vi "LSX Set Dig IO Distance.vi"(6 "lAxis":i32, 7 "dDist":dbl, 8 "error in (no error)":errorcluster, 9 "bFkt":i32, 10 "lIndex":i32, 11 "lLSID":i32) -> (0 "error out":errorcluster, 3 "function return":i32)   [LabVIEW 2016, in "Tango_DLL.lvlib"]
doc: "TANGOAPI int TANGOCALL LSX_SetDigIO_Distance (int lLSID, int lIndex, BOOL bFkt, double dDist, int lAxis);"
uses:
  Tango_DLL.lvlib
  2017/Microscope Control/Device Library/Stages/Marzhauser/SCAN IM 120 x 80/Tango DLL VIs/Tango_DLL.dll
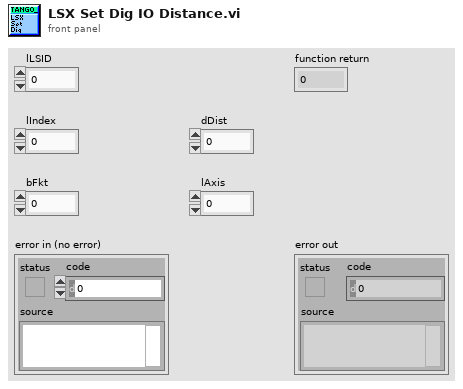
[diagram p1: front panel]
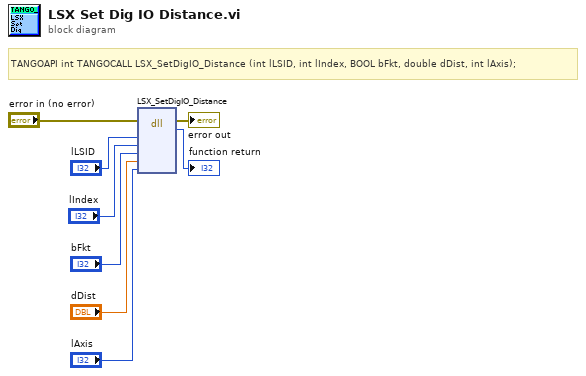
[diagram p0: block diagram]
diagram:
  # "TANGOAPI int TANGOCALL LSX_SetDigIO_Distance (int lLSID, int lIndex, BOOL bFkt, double dDist, int lAxis);"
  n1 = dll-call lib="C:/Users/4PiSMS/Documents/Microscope Control/2017/Microscope Control/Device Library/Stages/Marzhauser/SCAN IM 120 x 80/Tango DLL VIs/Tango_DLL.*" fn="LSX_SetDigIO_Distance"(error in="error in (no error)", "lLSID"="lLSID", "lIndex"="lIndex", "bFkt"="bFkt", "dDist"="dDist", "lAxis"="lAxis") -> (error out=→"error out":errorcluster, →"function return":i32)  [unwired: 7 in, 1 out]
